vi "Ctor.vi"(8 "error in (no error)":errorcluster) -> (0 "error out":errorcluster, 3 "LV Chat Server out":refnum<class "LV Chat Server.lvclass">)   [LabVIEW 2020, in "LV Chat Server.lvclass"]
uses:
  LV Chat Server.lvclass
  Ref Data.ctl
  User.ctl
  Stream-Simple-Msg/Endpoint/Endpoint.lvclass
  LV Chat Server.lvclass/LV Chat Server.ctl
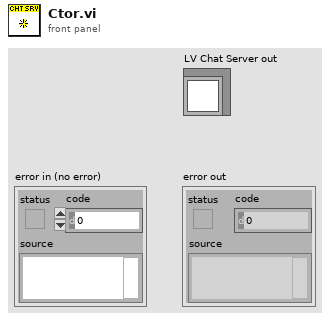
[diagram p1: front panel]
types:
  T1 = typedef "LV Chat Server.lvclass/Ref Data.ctl" = cluster{"Endpoint Map":map{string, T2}, "User Map":map{string, string}}
  T2 = typedef "LV Chat Server.lvclass/User.ctl" = cluster{"Name":string, "IP":string, "Connected At":dbl, "Endpoint":refnum<class "Endpoint.lvclass">}
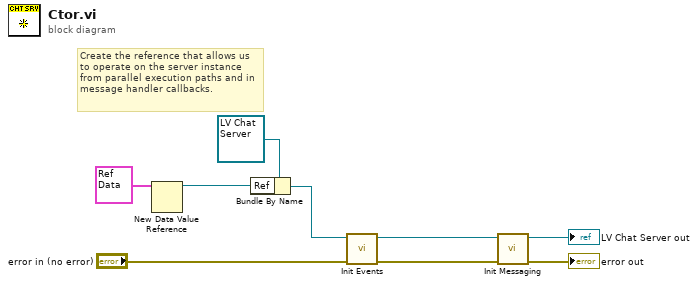
[diagram p0: block diagram]
diagram:
  # "Create the reference that allows us to operate on the server instance from parallel execution paths and in message handler callbacks."
  n1 = New Data Value Reference(data value=T1 {"Endpoint Map"={}, "User Map"={}} ("Ref Data")) -> (data value reference=w7:refnum<data-value>)  [unwired: 1 in, 1 out]
  n2 = Bundle By Name(cluster=refnum<class "LV Chat Server.lvclass"> refnum ("LV Chat Server in"), "Ref"=w7) -> (w2:refnum<class "LV Chat Server.lvclass">)
  n3 = call "Init Events.vi"("error in (no error)"="error in (no error)", "LV Chat Server in"=w2) -> ("error out"=w4:errorcluster, "LV Chat Server out"=w3:refnum<class "LV Chat Server.lvclass">)  [unwired: 8 in]
  n4 = call "Init Messaging.vi"("error in (no error)"=w4, "LV Chat Server in"=w3) -> ("error out"=→"error out":errorcluster, "LV Chat Server out"=→"LV Chat Server out":refnum<class "LV Chat Server.lvclass">)  [unwired: 8 in]
